vi "get async msg.vi"(10 "error in (no error)":errorcluster, 11 "Msg String in":string) -> (2 "error out":errorcluster, 3 "AsyncMsg":T1)   [LabVIEW 2019, in "Main.lvclass"]
doc: "Developed by Kevin Thompson\nkevin@thompsonengineering.net\n\nCopyright 2018\nThompson Engineering, LLC"
uses:
  Main.lvclass
  DataTypes/AsynMsg_Main--enum.ctl
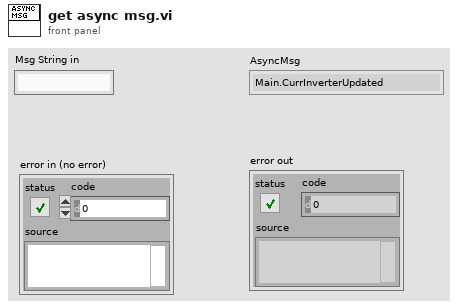
[diagram p1: front panel]
types:
  T1 = typedef "Main.lvclass/AsynMsg_Main--enum.ctl" = enum16{"Main.CurrInverterUpdated"}
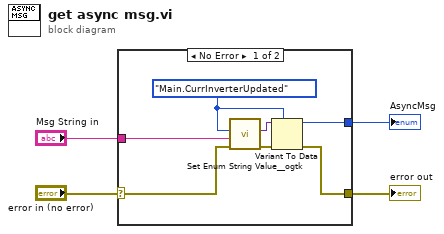
[diagram p0: block diagram]
diagram:
  n1 = case shown="No Error" "error in (no error)" {
    selector: "error in (no error)" -> [w6 w12]
    tunnel: "Msg String in" -> [w10 _]
    tunnel: [w9 _] -> w3
    tunnel: [w7 w12] -> w2
    frame No Error {
      w5 = AsynMsg_Main--enum."Main.CurrInverterUpdated" ("AsyncMsg")
      n2 = call <userlib>:"Set Enum String Value__ogtk.vi"("error in (no error)"=w6, "String Value"=w10, "Default Enum Value"=w5) -> ("error out"=w8:errorcluster, "Enum"=w11:variant)  [unwired: 7 in]
      n3 = Variant To Data(error in=w8, type=w5, Variant=w11) -> (data=w9:T1, error out=w7:errorcluster)
    }
    frame Error {
    }
  }
  "AsyncMsg" <- w3
  "error out" <- w2
